vi "Configure Session.vi"(8 "error in":errorcluster, 11 "Plugin in":refnum<class "StreamReader.lvclass">) -> (0 "error out":errorcluster, 3 "Plugin out":refnum<class "StreamReader.lvclass">)   [LabVIEW 2024, in "StreamReader.lvlib" / "StreamReader.lvclass"]
uses:
  StreamReader.lvclass
  C:/Program Files/National Instruments/LabVIEW 2024/vi.lib/FlexLogger/SDK/PluginSDK.lvlibp/PEFClasses/SDK/Plugin/Plugin.lvclass
  StreamReader.lvclass/StreamReader.ctl
  StreamReader Strings.vi
  <vilib>/FlexLogger/SDK/PluginSDK.lvlibp/PEFClasses/SDK/Plugin/ParameterAccess/Read String.vi
  <vilib>/FlexLogger/SDK/PluginSDK.lvlibp/PEFClasses/SDK/Plugin/ParameterAccess/Read I32.vi
  <vilib>/FlexLogger/SDK/PluginSDK.lvlibp/PEFClasses/SDK/Plugin/Plugin.lvclass
  C:/Program Files/National Instruments/LabVIEW 2024/vi.lib/FlexLogger/SDK/PluginSDK.lvlibp/PEFClasses/SDK/Processing Element/Processing Element.lvclass
  C:/dev/niflexlogger-plugins/plugins/StreamReader/source/StreamReader/StreamReader.lvclass
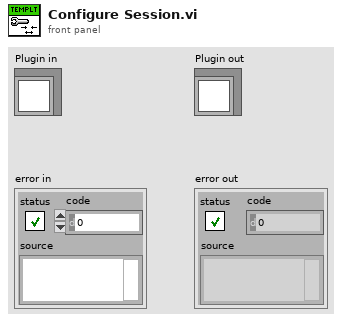
[diagram p1: front panel]
types:
  T1 = typedef "StreamReader.lvlib/StreamReader.lvclass/StreamReader Parameters.ctl" = cluster{"Reader URL":string, "Writer URL":string, "Buffer Size":i32, "Reader endpoint":refnum<k21>, "Channel Names":string[]}
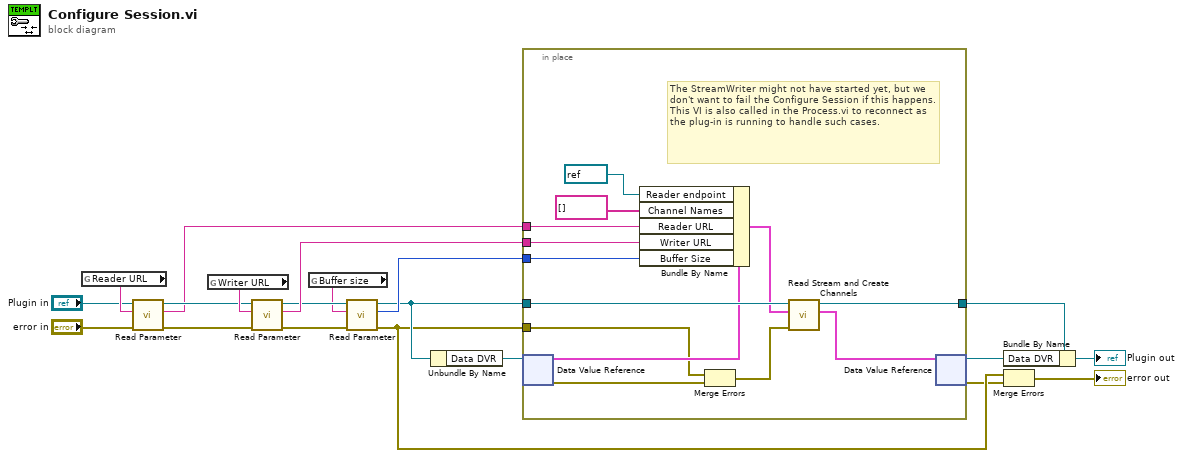
[diagram p0: block diagram]
diagram:
  n1 = global read "StreamReader Strings.vi" "Reader URL"() -> (w15:string)
  n2 = call-poly <vilib>:"Read Parameter.vi"("error in (no error)"="error in", "Name"=w15, "Plugin in"="Plugin in") -> ("error out"=w2:errorcluster, "Value"=w11:string, "Plugin out"=w13:refnum<class "StreamReader.lvclass">)  [unwired: 5 in, 1 out]
  n3 = global read "StreamReader Strings.vi" "Writer URL"() -> (w20:string)
  n4 = call-poly <vilib>:"Read Parameter.vi"("error in (no error)"=w2, "Name"=w20, "Plugin in"=w13) -> ("error out"=w4:errorcluster, "Value"=w17:string, "Plugin out"=w5:refnum<class "StreamReader.lvclass">)  [unwired: 5 in, 1 out]
  n5 = global read "StreamReader Strings.vi" "Buffer size"() -> (w3:string)
  n6 = call-poly <vilib>:"Read Parameter.vi"("error in (no error)"=w4, "Name"=w3, "Plugin in"=w5) -> ("error out"=w7:errorcluster, "Value"=w18:i32, "Plugin out"=w10:refnum<class "StreamReader.lvclass">)  [unwired: 5 in, 1 out]
  n7 = Unbundle By Name(w10) -> ("Data DVR"=w9:refnum<data-value>)
  n8 = in-place {
    in-place-border: w18 -> [w33]
    in-place-border: w17 -> [w32]
    in-place-border: w10 -> [w31]
    in-place-border: [w29] -> w16
    in-place-border: w7 -> [w24]
    in-place-border: w11 -> [w28]
    # "The StreamWriter might not have started yet, but we don't want to fail the Configure Session if this happens.\nThis VI is also called in the Process.vi to reconnect as the plug-in is running to handle such cases."
    n9 = in-place-dvr #1(w9) -> (w27:T1, w25:errorcluster)
    n10 = Bundle By Name(cluster=w27, "Reader endpoint"=refnum<k21> refnum, "Channel Names"=string[] [], "Reader URL"=w28, "Writer URL"=w32, "Buffer Size"=w33) -> (w30:T1)
    n11 = Merge Errors(w24, w25) -> (w23:errorcluster)
    n12 = call-dynamic "Read Stream and Create Channels.vi"("error in (no error)"=w23, "StreamReader Parameters in"=w30, "Plugin in"=w31) -> ("StreamReader Parameters out"=w26:T1, "Plugin out"=w29:refnum<class "StreamReader.lvclass">)  [unwired: 5 in, 2 out]
    n13 = in-place-dvr #1(w26) -> (w8:refnum<data-value>, w6:errorcluster)
  }
  n14 = Bundle By Name(cluster=w16, "Data DVR"=w8) -> (→"Plugin out":refnum<class "StreamReader.lvclass">)
  n15 = Merge Errors(w7, w6) -> (→"error out":errorcluster)
